vi "Speed of VIght FPGA.vi"() -> ()   [LabVIEW 2025]
uses:
  <vilib>/eio/EIONode/EIONode.xnode
  <vilib>/rvi/eio/common/nirviEmuTemplateMethod_errors.vi
panel:
  out "Player 2 Bonus":u8
  out "Player 1 Bonus":u8
  in  "Max Bonus":u8=5
  in  "Bonus Threshold":u64=3000
  out "Intial Random Arrays":u8[](array[numeric])
  out "Player2 Input":bool[](array[boolean])
  out "Player1 Input":bool[](array[boolean])
  out "Player 2 Output 4":bool[](array[boolean])
  out "Player 2 Output 3":bool[](array[boolean])
  out "Player 2 Output 2":bool[](array[boolean])
  out "Player 2 Output 1":bool[](array[boolean])
  out "Player 1 Output 4":bool[](array[boolean])
  out "Player 1 Output 3":bool[](array[boolean])
  out "Player 1 Output 2":bool[](array[boolean])
  out "Player 2 Score":u32
  out "Player 2 Timer":u64
  out "Player 1 Score":u32
  out "Player 1 Timer":u64
  out "Main Loop":i32
  out "Closing Loop":i32
  out "Element to change 2":i32
  out "Element to change":i32
  out "Measured Main Loop Ticks":u32
  in  "Main Loop Timer":u32=1 caption="Main Loop Timer (uSec)"
  out "Player2 Output Number":u32
  out "Player1 Output Number":u32
  out "Initialized Array 2":bool[](array[boolean])
  out "Initialized Array 1":bool[](array[boolean])
  out "Random Number":u8
  in  "Random Number Max":u8=20
  out "Idle Loop":i32
  out "Current State":i16
  out "Blue2":bool
  out "Green3":bool
  out "Green2":bool
  out "Blue1":bool
  out "Green1":bool
  out "Player 1 Output":bool[](array[boolean])
  in  "Game Length (s)":u32=45
  in  "Stop Closing Loop":bool
  in  "Stop Main Loop":bool
  in  "Stop Idle":bool
  in  "Global Stop":bool
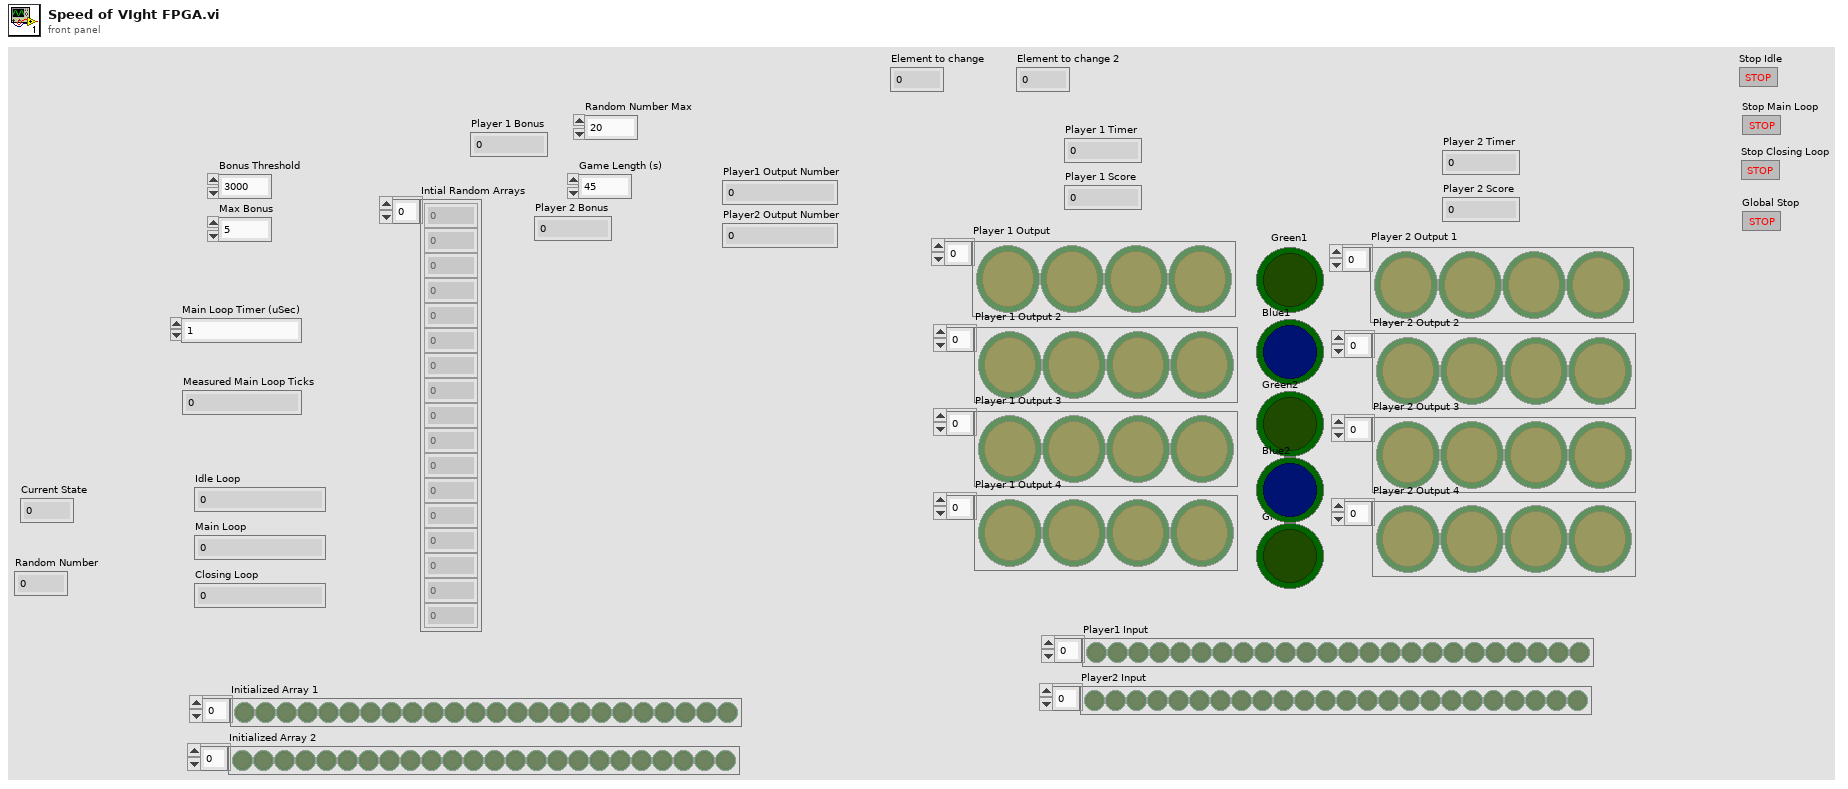
[diagram p1: front panel]
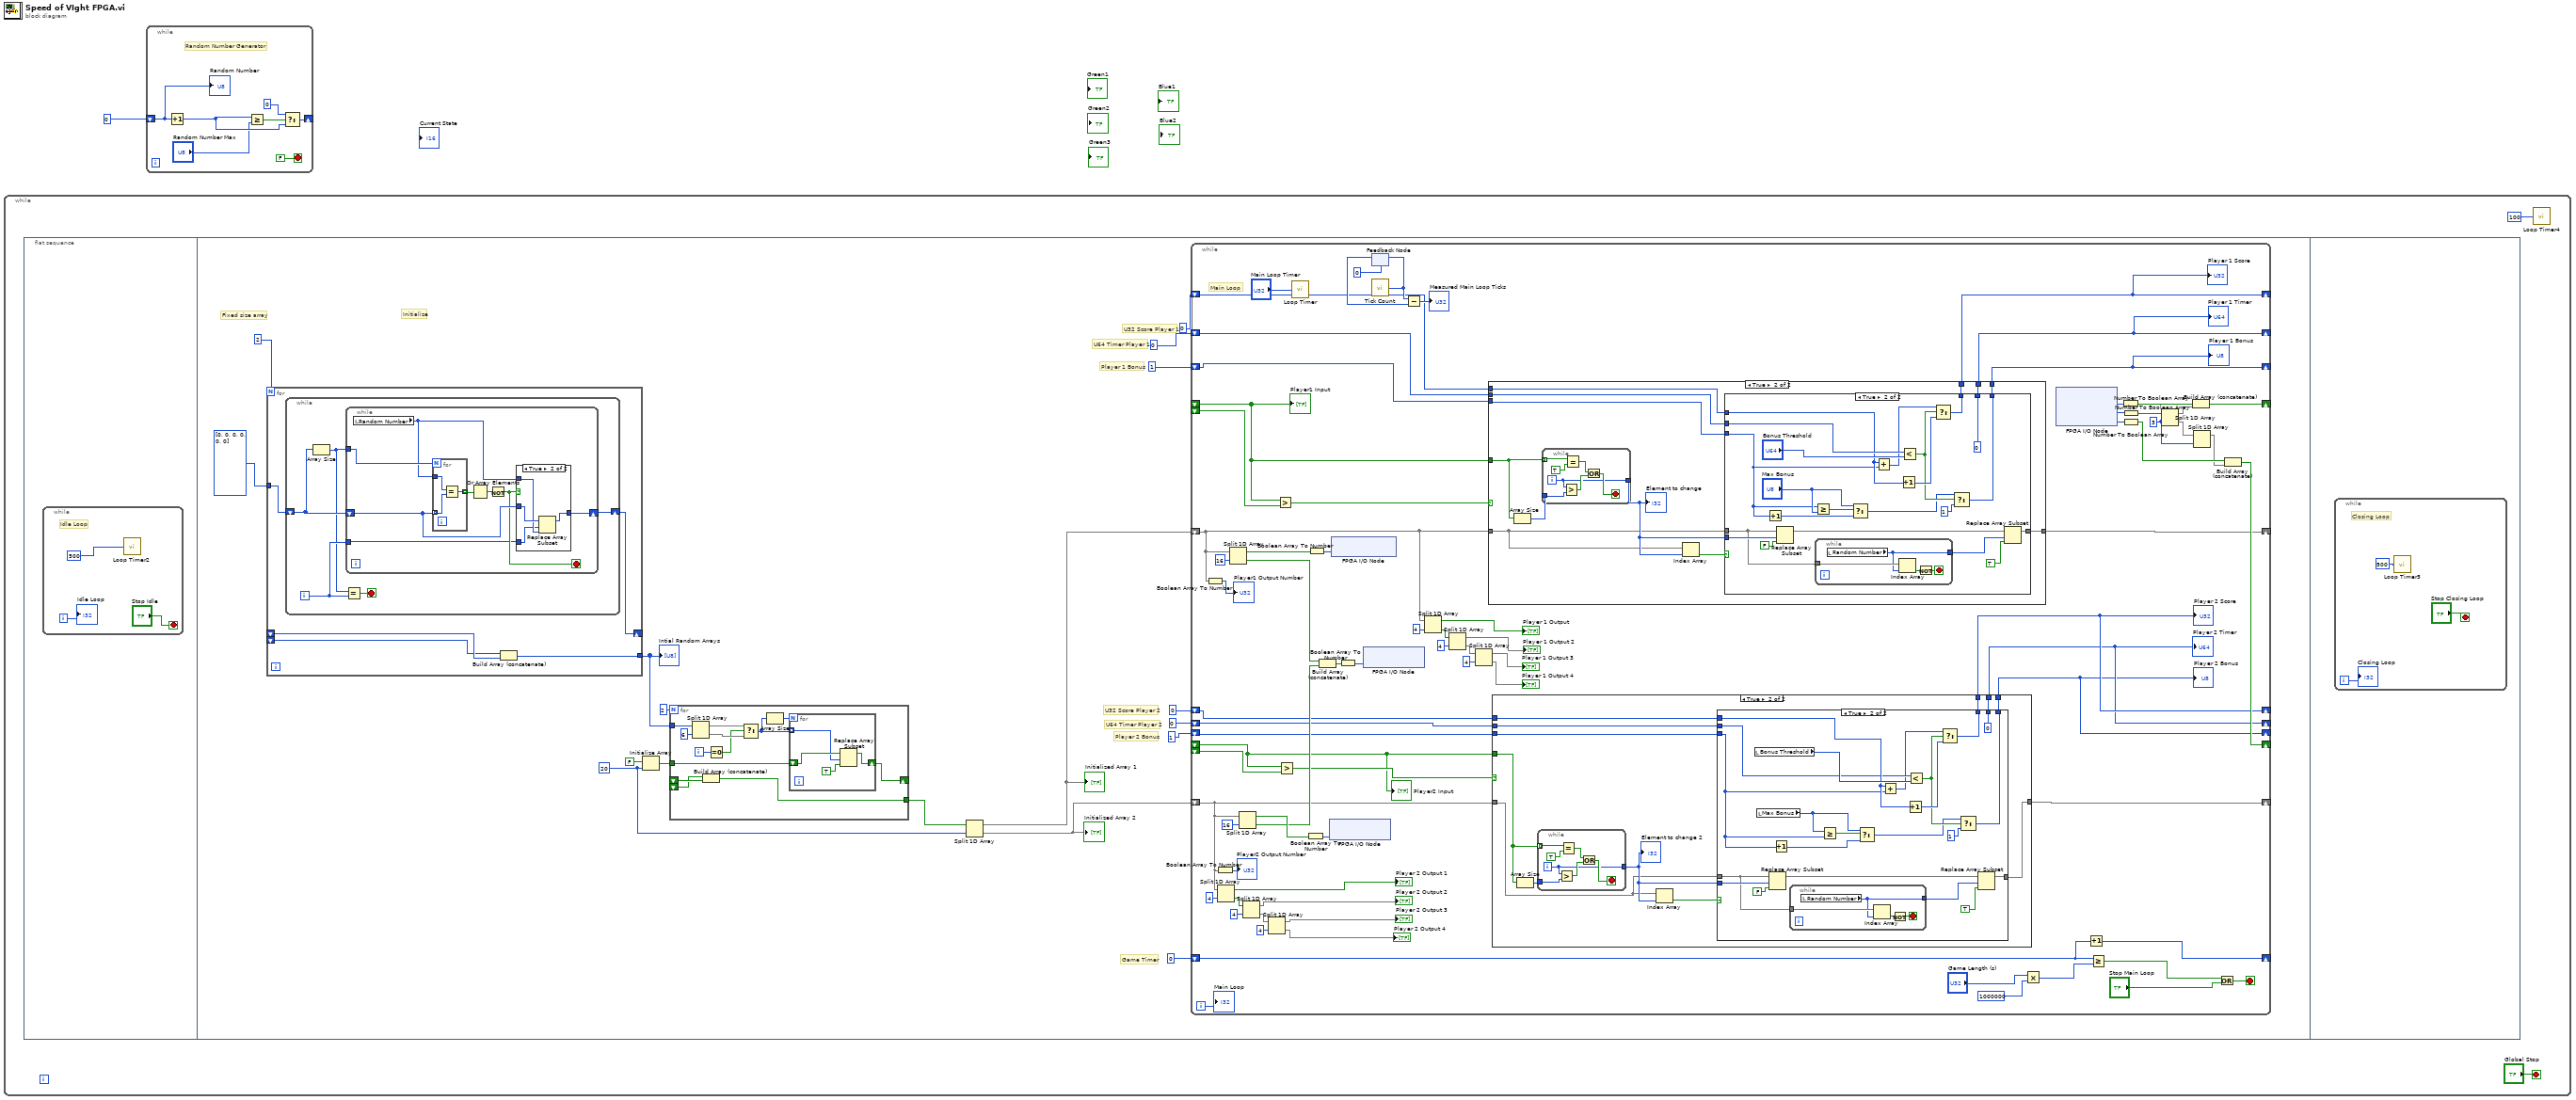
[diagram p0: block diagram]
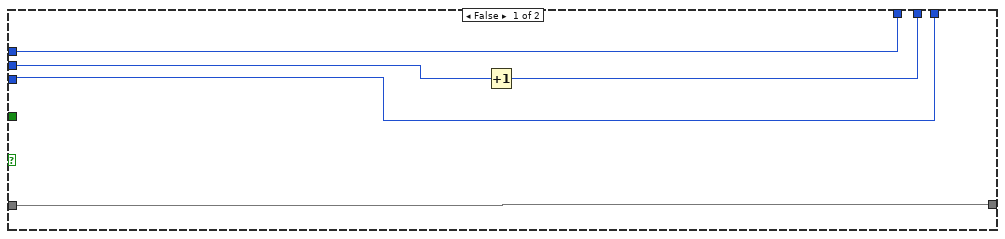
[diagram p3: hidden frame]
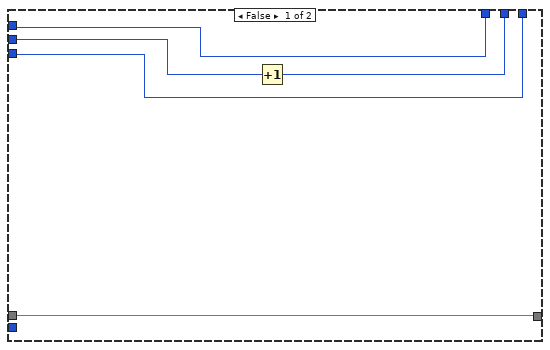
[diagram p4: hidden frame]
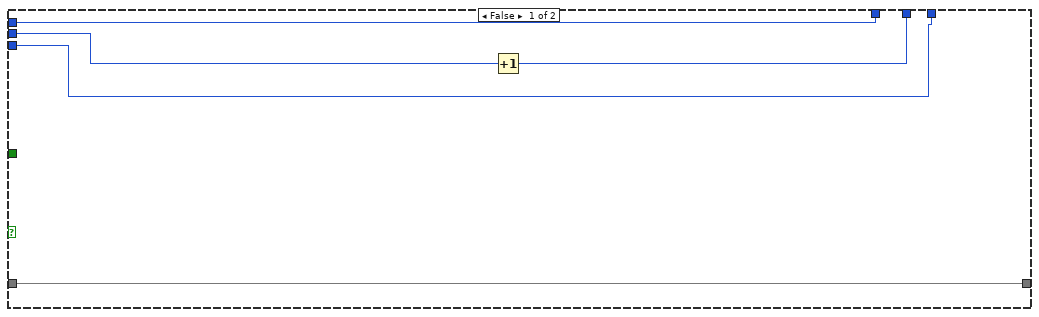
[diagram p5: hidden frame]
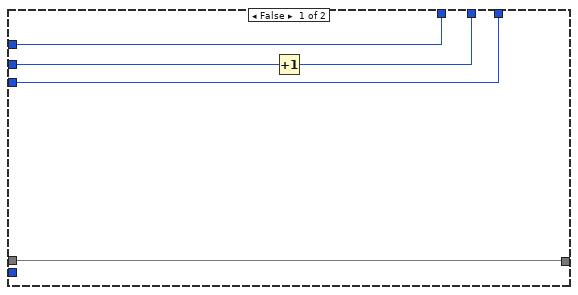
[diagram p6: hidden frame]
diagram:
  n1 = while {
    stop <- "Global Stop" stop-if-true
    n2 = flat-sequence {
      frame #0 {
        n3 = while {
          i -> [w5]
          stop <- "Stop Idle" stop-if-true
          # "Idle Loop"
          n4 = call "Loop Timer2"("Count(mSec)"=u32 500 ("millisecond multiple")) -> ()  [unwired: 1 out]
          "Idle Loop" <- w5
        }
      }
      frame #1 {
        w10 = 20 ("dimension size")
        # "Player 2 Bonus"
        # "Player 1 Bonus"
        # "Initialize"
        # "Fixed size array"
        # "Game Timer"
        # "U32 Score Player 2"
        # "U32 Score Player 1"
        # "U64 Timer Player 2"
        # "U64 Timer Player 1"
        n5 = for {
          N: 2 -> [_]
          tunnel: u8[] [0, 0, 0, 0, 0, 0] ("Initial Random Numbers") -> [w45]
          shift-right: [w44] -> _
          shift-left: _ -> [w43]
          shift-left: _ -> [w42]
          tunnel: [w41] -> w13
          n6 = while {
            shift-right: [w46] -> w44
            shift-left: w45 -> [w48]
            i -> [w50]
            stop <- w49 stop-if-true
            n7 = Array Size(array=w48) -> (size(s)=w47:i32)
            n8 = Equal?(x=w47, y=w50) -> (x = y?=w49:bool)
            n9 = while {
              tunnel: w50 -> [w52]
              shift-right: [w53] -> w46
              shift-left: w48 -> [w55]
              tunnel: w47 -> [w58]
              stop <- w54 stop-if-true
              n10 = local read "Random Number"() -> (w51:u8)
              n11 = for {
                N: w58 -> [_]
                tunnel: w55 -> [w65] mode=indexing
                tunnel: w51 -> [w66]
                tunnel: [w64] -> w57 mode=indexing
                n12 = Equal?(x=w66, y=w65) -> (x = y?=w64:bool)
              }
              n13 = Or Array Elements(Boolean array=w57) -> (logical OR=w56:bool)
              n14 = Not(x=w56) -> (.not. x?=w54:bool)
              n15 = case shown="True" w54 {
                tunnel: w55 -> [w59 w63]
                tunnel: [w59 w62] -> w53
                tunnel: w51 -> [_ w61]
                tunnel: w52 -> [_ w60]
                frame False {
                }
                frame True {
                  n16 = Replace Array Subset(array=w63, new element=w61, index=w60) -> (w62:u8[])
                }
              }
            }
          }
          n17 = Build Array (concatenate)(w42, w43) -> (w41:u8[])
        }
        "Intial Random Arrays" <- w13
        n18 = Initialize Array(FALSE ("Boolean"), w10) -> (w15:bool[])
        n19 = for {
          N: 2 -> [_]
          tunnel: w15 -> [w35]
          tunnel: w13 -> [w33]
          shift-right: [w36] -> _
          shift-left: _ -> [w26]
          shift-left: _ -> [w25]
          tunnel: [w24] -> w9
          i -> [w29]
          n20 = Split 1D Array(array=w33, index=6) -> (first subarray=w30:u8[], second subarray=w31:u8[])
          n21 = Build Array (concatenate)(w25, w26) -> (w24:bool[])
          n22 = Equal To 0?(x=w29) -> (x = 0?=w28:bool)
          n23 = Select(t=w30, s=w28, f=w31) -> (s? t:f=w27:u8[])
          n24 = Array Size(array=w27) -> (size(s)=w34:i32)
          n25 = for {
            N: w34 -> [_]
            tunnel: w27 -> [w37] mode=indexing
            shift-right: [w40] -> w36
            shift-left: w35 -> [w39]
            n26 = Replace Array Subset(array=w39, new element=TRUE ("new element/subarray"), index=w37) -> (w40:bool[])
          }
        }
        n27 = Split 1D Array(array=w9, index=w10) -> (first subarray=w12:bool[], second subarray=w11:bool[])
        "Initialized Array 1" <- w12
        "Initialized Array 2" <- w11
        n28 = while {
          shift-right: [w74] -> _
          shift-left: u64 0 -> [w78]
          shift-right: [w68] -> _
          shift-left: u64 0 -> [w72]
          shift-right: [w76] -> _
          shift-left: u32 0 -> [w77]
          shift-right: [w69] -> _
          shift-left: u32 0 -> [w70]
          shift-right: [w142] -> _
          shift-left: u32 0 -> [w143]
          shift-right: [w110] -> _
          shift-left: w12 -> [w85]
          shift-right: [w107] -> _
          shift-left: w11 -> [w99]
          shift-right: [w115] -> _
          shift-left: _ -> [w80]
          shift-right: [w114] -> _
          shift-left: _ -> [w79]
          shift-left: _ -> [w113]
          shift-left: _ -> [w109]
          shift-right: [w73] -> _
          shift-left: u8 1 -> [w75]
          shift-right: [w67] -> _
          shift-left: u8 1 -> [w71]
          i -> [w102]
          stop <- w106 stop-if-true
          w121 = 3 ("index")
          # "Main Loop"
          n29 = Boolean Array To Number(Boolean array=w85) -> (number=→"Player1 Output Number":u32)
          n30 = Boolean Array To Number(Boolean array=w99) -> (number=→"Player2 Output Number":u32)
          n31 = Split 1D Array(array=w99, index=4) -> (first subarray=→"Player 2 Output 1":bool[], second subarray=w95:bool[])
          n32 = Split 1D Array(array=w85, index=16) -> (first subarray=w111:bool[], second subarray=w133:bool[])
          n33 = Split 1D Array(array=w99, index=16) -> (first subarray=w136:bool[], second subarray=w132:bool[])
          n34 = Split 1D Array(array=w95, index=4) -> (first subarray=→"Player 2 Output 2":bool[], second subarray=w93:bool[])
          n35 = Split 1D Array(array=w93, index=4) -> (first subarray=→"Player 2 Output 3":bool[], second subarray=→"Player 2 Output 4":bool[])
          n36 = Greater?(x=w80, y=w113) -> (0:w112:bool)
          n37 = Greater?(x=w79, y=w109) -> (0:w108:bool)
          n38 = call "Loop Timer"("Count(uSec)"="Main Loop Timer") -> ()  [unwired: 1 out]
          n39 = Boolean Array To Number(Boolean array=w136) -> (number=w135:u32)
          n40 = Boolean Array To Number(Boolean array=w111) -> (number=w138:u32)
          n41 = Build Array (concatenate)(w133, w132) -> (w131:bool[])
          n42 = xnode "FPGA I/O Node"("Mod8/DO7:0"=w135) -> ()  [unwired: 1 in, 1 out]
          n43 = xnode "FPGA I/O Node"("Mod6/DO15:0"=w138) -> ()  [unwired: 1 in, 1 out]
          n44 = Boolean Array To Number(Boolean array=w131) -> (number=w130:u32)
          n45 = xnode "FPGA I/O Node"("Mod7/DO7:0"=w130) -> ()  [unwired: 1 in, 1 out]
          n46 = feedback #1(u32 0) -> (w118:u32)
          n47 = call "Tick Count"() -> ("Tick Count(Ticks)"=w117:u32)
          n48 = feedback-in #1(w117) -> ()
          n49 = Subtract(x=w117, y=w118) -> (x-y=→"Measured Main Loop Ticks":u32)
          n50 = Split 1D Array(array=w85, index=4) -> (first subarray=→"Player 1 Output":bool[], second subarray=w87:bool[])
          n51 = Split 1D Array(array=w87, index=4) -> (first subarray=→"Player 1 Output 2":bool[], second subarray=w86:bool[])
          n52 = Split 1D Array(array=w86, index=4) -> (first subarray=→"Player 1 Output 3":bool[], second subarray=→"Player 1 Output 4":bool[])
          n53 = case shown="True" w112 {
            tunnel: [w204 w216] -> w110
            tunnel: w80 -> [_ w213]
            tunnel: w85 -> [w204 w211]
            tunnel: w78 -> [w202 w207]
            tunnel: [w201 w209] -> w74
            tunnel: w77 -> [w203 w208]
            tunnel: [w203 w210] -> w76
            tunnel: w75 -> [w200 w206]
            tunnel: [w200 w205] -> w73
            frame False {
              n54 = Increment(x=w202) -> (x+1=w201:u64)
            }
            frame True {
              n55 = Array Size(array=w213) -> (size(s)=w212:i32)
              n56 = while {
                tunnel: w213 -> [w254] mode=indexing
                tunnel: w212 -> [w250]
                tunnel: [w248] -> w215
                i -> [w248]
                stop <- w251 stop-if-true
                n57 = Greater?(x=w248, y=w250) -> (0:w249:bool)
                n58 = Equal?(x=w254, y=TRUE ("element")) -> (x = y?=w252:bool)
                n59 = Or(x=w252, y=w249) -> (x .or. y?=w251:bool)
              }
              "Element to change" <- w215
              n60 = Index Array(array=w211, index=w215) -> (element=w214:bool)
              n61 = case shown="True" w214 {
                tunnel: w215 -> [_ w243]
                tunnel: [w221 w239] -> w216
                tunnel: w211 -> [w221 w237]
                tunnel: w208 -> [w220 w224]
                tunnel: w207 -> [w219 w235]
                tunnel: [w220 w233] -> w210
                tunnel: [w218 u64 0] -> w209
                tunnel: w206 -> [w217 w223]
                tunnel: [w217 w230] -> w205
                frame False {
                  n62 = Increment(x=w219) -> (x+1=w218:u64)
                }
                frame True {
                  n63 = Increment(x=w223) -> (x+1=w226:u8)
                  n64 = Replace Array Subset(array=w237, new element=FALSE ("new element/subarray"), index=w243) -> (w241:bool[])
                  n65 = Greater Or Equal?(x=w223, y="Max Bonus") -> (x >= y?=w228:bool)
                  n66 = while {
                    tunnel: [w244] -> w238
                    tunnel: w237 -> [w247]
                    stop <- w245 stop-if-true
                    n67 = local read "Random Number"() -> (w244:u8)
                    n68 = Index Array(array=w247, index=w244) -> (element=w246:bool)
                    n69 = Not(x=w246) -> (.not. x?=w245:bool)
                  }
                  n70 = Select(t="Max Bonus", s=w228, f=w226) -> (s? t:f=w225:u8)
                  n71 = Add(x=w224, y=w223) -> (x+y=w222:u32)
                  n72 = Increment(x=w224) -> (x+1=w234:u32)
                  n73 = Less?(x=w235, y="Bonus Threshold") -> (x < y?=w232:bool)
                  n74 = Select(t=w222, s=w232, f=w234) -> (s? t:f=w233:u32)
                  n75 = Select(t=w225, s=w232, f=u8 1) -> (s? t:f=w230:u8)
                  n76 = Replace Array Subset(array=w241, new element=TRUE ("new element/subarray"), index=w238) -> (w239:bool[])
                }
              }
            }
          }
          "Player 1 Timer" <- w74
          "Player 1 Score" <- w76
          "Player 1 Bonus" <- w73
          n77 = case shown="True" w108 {
            tunnel: [w149 w157] -> w107
            tunnel: w79 -> [_ w159]
            tunnel: w99 -> [w149 w156]
            tunnel: w72 -> [w147 w154]
            tunnel: w71 -> [w145 w153]
            tunnel: w70 -> [w148 w155]
            tunnel: [w148 w151] -> w69
            tunnel: [w146 w152] -> w68
            tunnel: [w145 w150] -> w67
            frame False {
              n78 = Increment(x=w147) -> (x+1=w146:u64)
            }
            frame True {
              n79 = Array Size(array=w159) -> (size(s)=w158:i32)
              n80 = while {
                tunnel: w159 -> [w199] mode=indexing
                tunnel: w158 -> [w195]
                tunnel: [w193] -> w161
                i -> [w193]
                stop <- w196 stop-if-true
                n81 = Greater?(x=w193, y=w195) -> (0:w194:bool)
                n82 = Equal?(x=w199, y=TRUE ("element")) -> (x = y?=w197:bool)
                n83 = Or(x=w197, y=w194) -> (x .or. y?=w196:bool)
              }
              "Element to change 2" <- w161
              n84 = Index Array(array=w156, index=w161) -> (element=w160:bool)
              n85 = case shown="True" w160 {
                tunnel: w161 -> [_ w188]
                tunnel: [w166 w184] -> w157
                tunnel: w156 -> [w166 w182]
                tunnel: w155 -> [w162 w174]
                tunnel: w154 -> [w165 w169]
                tunnel: w153 -> [w163 w167]
                tunnel: [w164 u64 0] -> w152
                tunnel: [w163 w172] -> w150
                tunnel: [w162 w171] -> w151
                frame False {
                  n86 = Increment(x=w165) -> (x+1=w164:u64)
                }
                frame True {
                  n87 = local read "Bonus Threshold"() -> (w176:u64)
                  n88 = local read "Max Bonus"() -> (w175:u8)
                  n89 = Replace Array Subset(array=w182, new element=FALSE ("new element/subarray"), index=w188) -> (w186:bool[])
                  n90 = Increment(x=w167) -> (x+1=w170:u8)
                  n91 = while {
                    tunnel: [w189] -> w183
                    tunnel: w182 -> [w192]
                    stop <- w190 stop-if-true
                    n92 = local read "Random Number"() -> (w189:u8)
                    n93 = Index Array(array=w192, index=w189) -> (element=w191:bool)
                    n94 = Not(x=w191) -> (.not. x?=w190:bool)
                  }
                  n95 = Greater Or Equal?(x=w175, y=w167) -> (x >= y?=w178:bool)
                  n96 = Select(t=w175, s=w178, f=w170) -> (s? t:f=w177:u8)
                  n97 = Add(x=w174, y=w167) -> (x+y=w168:u32)
                  n98 = Increment(x=w174) -> (x+1=w181:u32)
                  n99 = Less?(x=w169, y=w176) -> (x < y?=w180:bool)
                  n100 = Select(t=w168, s=w180, f=w181) -> (s? t:f=w171:u32)
                  n101 = Select(t=w177, s=w180, f=u8 1) -> (s? t:f=w172:u8)
                  n102 = Replace Array Subset(array=w186, new element=TRUE ("new element/subarray"), index=w183) -> (w184:bool[])
                }
              }
            }
          }
          "Player 2 Timer" <- w68
          "Player 2 Score" <- w69
          "Player 2 Bonus" <- w67
          n103 = Multiply(x="Game Length (s)", y=u32 1000000) -> (x*y=w103:u32)
          n104 = xnode "FPGA I/O Node"() -> ("Mod6/DI15:0"=w129:u16, "Mod7/DI15:0"=w128:u16, "Mod8/DI15:0"=w127:u16)  [unwired: 3 in, 3 out]
          n105 = Increment(x=w143) -> (x+1=w142:u32)
          n106 = Greater Or Equal?(x=w143, y=w103) -> (x >= y?=w141:bool)
          n107 = Number To Boolean Array(number=w129) -> (Boolean array=w124:bool[])
          n108 = Number To Boolean Array(number=w128) -> (Boolean array=w125:bool[])
          n109 = Number To Boolean Array(number=w127) -> (Boolean array=w122:bool[])
          n110 = Split 1D Array(array=w125, index=w121) -> (first subarray=w123:bool[], second subarray=w120:bool[])
          n111 = Build Array (concatenate)(w124, w123) -> (w115:bool[])
          n112 = Split 1D Array(array=w120, index=w121) -> (first subarray=w119:bool[])  [unwired: 1 out]
          n113 = Or(x=w141, y="Stop Main Loop") -> (x .or. y?=w106:bool)
          n114 = Build Array (concatenate)(w122, w119) -> (w114:bool[])
          "Main Loop" <- w102
          "Player1 Input" <- w80
          "Player2 Input" <- w79
        }
      }
      frame #2 {
        n115 = while {
          i -> [w256]
          stop <- "Stop Closing Loop" stop-if-true
          # "Closing Loop"
          n116 = call "Loop Timer3"("Count(mSec)"=u32 500 ("millisecond multiple")) -> ()  [unwired: 1 out]
          "Closing Loop" <- w256
        }
      }
    }
    n117 = call "Loop Timer4"("Count(mSec)"=u32 100 ("millisecond multiple")) -> ()  [unwired: 1 out]
  }
  n118 = while {
    shift-right: [w261] -> _
    shift-left: u8 0 -> [w263]
    stop <- FALSE stop-if-true
    # "Random Number Generator"
    n119 = Increment(x=w263) -> (x+1=w260:u8)
    n120 = Greater Or Equal?(x=w260, y="Random Number Max") -> (x >= y?=w259:bool)
    n121 = Select(t=u8 0, s=w259, f=w260) -> (s? t:f=w261:u8)
    "Random Number" <- w263
  }
